vi "Which Thumbnail.vi"(8 "error in (no error)":errorcluster, 10 "Coords":T1, 11 "[Thumbnails]":T2[](array[typedef])) -> (0 "error out":errorcluster, 2 "Path":path, 3 "index of element":i32)   [LabVIEW 2018]
uses:
  Thumbnail Cluster.ctl
  <vilib>/Utility/miscctls.llb/LVPoint32TypeDef.ctl
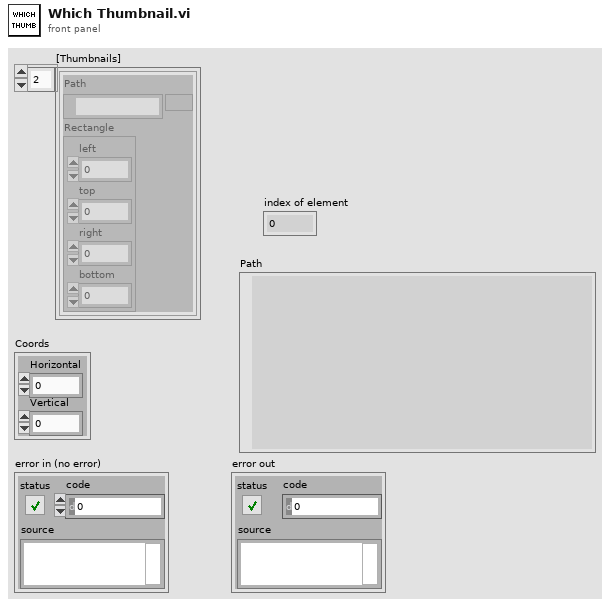
[diagram p1: front panel]
types:
  T1 = typedef "LVPoint32TypeDef.ctl" = cluster{"Horizontal":i32, "Vertical":i32}
  T2 = typedef "Thumbnail Cluster.ctl" = cluster{"Path":path, "Rectangle":cluster{"left":i16, "top":i16, "right":i16, "bottom":i16}}
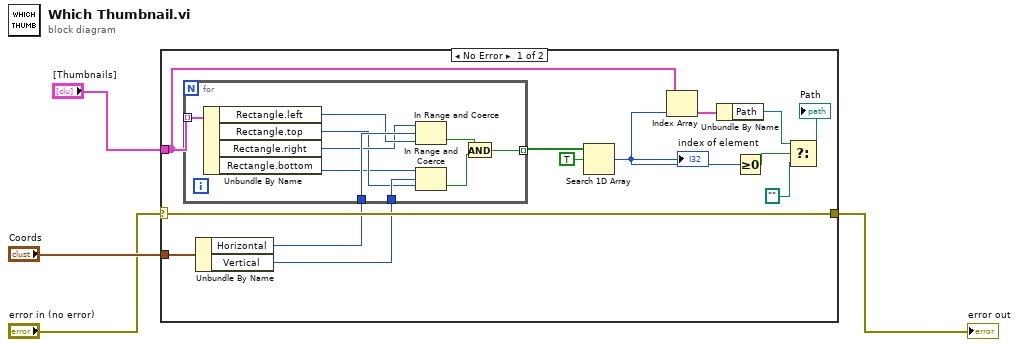
[diagram p0: block diagram]
diagram:
  n1 = case shown="No Error" "error in (no error)" {
    selector: "error in (no error)" -> [w17 w28]
    tunnel: [w17 w28] -> w2
    tunnel: "Coords" -> [w16 _]
    tunnel: "[Thumbnails]" -> [w11 _]
    frame No Error {
      n2 = Unbundle By Name(w16) -> ("Horizontal"=w15:i32, "Vertical"=w14:i32)
      n3 = for {
        tunnel: w11 -> [w27] mode=indexing
        tunnel: w15 -> [w26]
        tunnel: w14 -> [w23]
        tunnel: [w18] -> w13 mode=indexing
        n4 = Unbundle By Name(w27) -> ("Rectangle.left"=w25:i16, "Rectangle.top"=w22:i16, "Rectangle.right"=w24:i16, "Rectangle.bottom"=w21:i16)
        n5 = In Range and Coerce(upper limit=w24, x=w26, lower limit=w25) -> (In Range?=w20:bool)  [unwired: 1 out]
        n6 = In Range and Coerce(upper limit=w21, x=w23, lower limit=w22) -> (In Range?=w19:bool)  [unwired: 1 out]
        n7 = And(x=w20, y=w19) -> (x .and. y?=w18:bool)
      }
      n8 = Search 1D Array(1D array=w13, element=TRUE) -> (index of element=w9:i32)  [unwired: 1 in]
      "index of element" <- w9
      n9 = Index Array(array=w11, index=w9) -> (element=w10:T2)
      n10 = Unbundle By Name(w10) -> ("Path"=w7:path)
      n11 = Greater Or Equal To 0?(x=w9) -> (x >= 0?=w8:bool)
      n12 = Select(t=w7, s=w8, f=path "") -> (s? t:f=→"Path":path)
    }
    frame Error {
    }
  }
  "error out" <- w2
